vi "main_run.vi"(6 "Cleanup?":refnum<vi>, 7 "Running?":refnum<vi>, 8 "Stop Button":refnum<vi>, 9 "Pause Button":refnum<vi>, 10 "Reset":refnum<vi>, 11 "Run":refnum<vi>) -> ()   [LabVIEW 2019]
panel:
  # "*******************************************************************\nBiogas Plant Control\n\nAuthor: Paul Zügel\nGCSC-Frankfurt am Main 2020\n\n*******************************************************************"
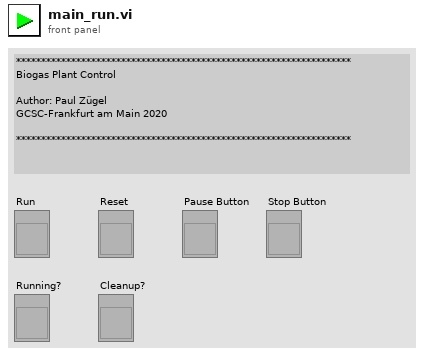
[diagram p1: front panel]
types:
  T1 = enum8{"Enabled", "Disabled", "Disabled and Grayed Out"}
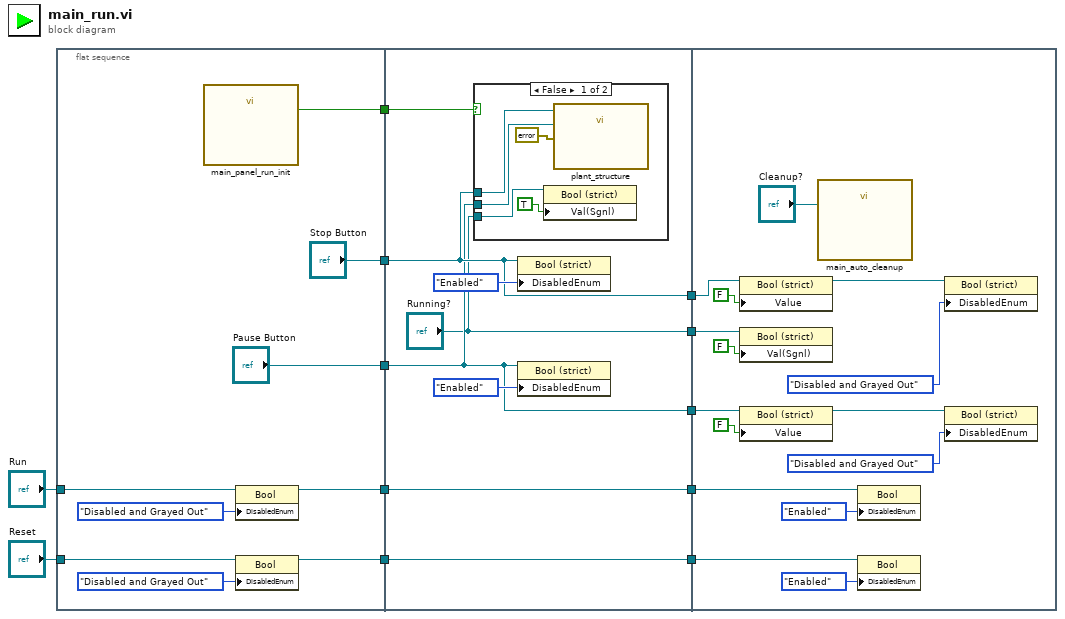
[diagram p0: block diagram]
diagram:
  n1 = flat-sequence {
    tunnel: "Run" -> [w19]
    tunnel: "Reset" -> [w18]
    tunnel: [w17] -> w8
    tunnel: [w16] -> w6
    tunnel: ["Pause Button"] -> w4
    tunnel: ["Stop Button"] -> w3
    tunnel: [w13] -> w2
    tunnel: [w24] -> w11
    tunnel: [w23] -> w9
    tunnel: w8 -> [w29]
    tunnel: [w29] -> w7
    tunnel: w6 -> [w28]
    tunnel: [w28] -> w5
    tunnel: w4 -> [w23]
    tunnel: w3 -> [w24]
    tunnel: w2 -> [w25]
    tunnel: ["Running?"] -> w1
    tunnel: w11 -> [w46]
    tunnel: w9 -> [w39]
    tunnel: w7 -> [w41]
    tunnel: w5 -> [w40]
    tunnel: w1 -> [w36]
    frame #0 {
      n2 = call "main_panel_run_init.vi"() -> ("Cancelled?"=w13:bool)  [unwired: 3 in]
      n3 = property on="Property Node" class="Bool"(reference=w19, "DisabledEnum"=T1."Disabled and Grayed Out" ("Disabled")) -> (reference out=w17:refnum<vi>)  [unwired: 1 in, 1 out]
      n4 = property on="Property Node" class="Bool"(reference=w18, "DisabledEnum"=T1."Disabled and Grayed Out" ("Disabled")) -> (reference out=w16:refnum<vi>)  [unwired: 1 in, 1 out]
    }
    frame #1 {
      n5 = case shown="False" w25 {
        tunnel: w24 -> [w33 _]
        tunnel: w23 -> [w32 _]
        tunnel: "Running?" -> [w31 _]
        frame False {
          n6 = property on="Property Node" class="Bool (strict)"(reference=w31, "Val(Sgnl)"=TRUE ("Value (Signaling)")) -> ()  [unwired: 1 in, 2 out]
          n7 = call "plant_structure.vi"("Dataflow"=errorcluster {"status"=FALSE, "code"=0, "source"=""}, "Pause"=w32, "Stop"=w33) -> ()  [unwired: 9 in]
        }
        frame True {
        }
      }
      n8 = property on="Property Node" class="Bool (strict)"(reference=w24, "DisabledEnum"=T1."Enabled" ("Disabled")) -> ()  [unwired: 1 in, 2 out]
      n9 = property on="Property Node" class="Bool (strict)"(reference=w23, "DisabledEnum"=T1."Enabled" ("Disabled")) -> ()  [unwired: 1 in, 2 out]
    }
    frame #2 {
      n10 = property on="Property Node" class="Bool (strict)"(reference=w46, "Value"=FALSE) -> (reference out=w37:refnum<vi>)  [unwired: 1 in, 1 out]
      n11 = property on="Property Node" class="Bool (strict)"(reference=w36, "Val(Sgnl)"=FALSE ("Value (Signaling)")) -> ()  [unwired: 1 in, 2 out]
      n12 = property on="Property Node" class="Bool (strict)"(reference=w39, "Value"=FALSE ("Stop Button")) -> (reference out=w38:refnum<vi>)  [unwired: 1 in, 1 out]
      n13 = call "main_auto_cleanup.vi"("Cleanup?"="Cleanup?") -> ()  [unwired: 11 in]
      n14 = property class="Bool"(reference=w41, "DisabledEnum"=T1."Enabled" ("Disabled")) -> ()  [unwired: 1 in, 2 out]
      n15 = property on="Property Node" class="Bool"(reference=w40, "DisabledEnum"=T1."Enabled" ("Disabled")) -> ()  [unwired: 1 in, 2 out]
      n16 = property class="Bool (strict)"(reference=w37, "DisabledEnum"=T1."Disabled and Grayed Out" ("Disabled")) -> ()  [unwired: 1 in, 2 out]
      n17 = property class="Bool (strict)"(reference=w38, "DisabledEnum"=T1."Disabled and Grayed Out" ("Disabled")) -> ()  [unwired: 1 in, 2 out]
    }
  }
